vi "RunOperation.vi"(10 "Inputs":string[](array[string]), 11 "Restore in":refnum<class "Restore.lvclass">) -> (1 "Output/Failure":string, 2 "CLI Process Return Code":i32, 3 "Restore out":refnum<class "Restore.lvclass">)   [LabVIEW 2017, in "Restore.lvclass"]
uses:
  Restore.lvclass
  Restore.lvclass/Restore.ctl
  <vilib>/JKI/VIPM API/VIPM API_vipm_api.lvlib
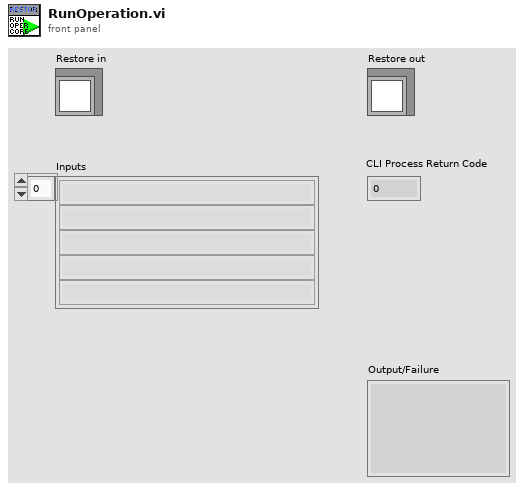
[diagram p1: front panel]
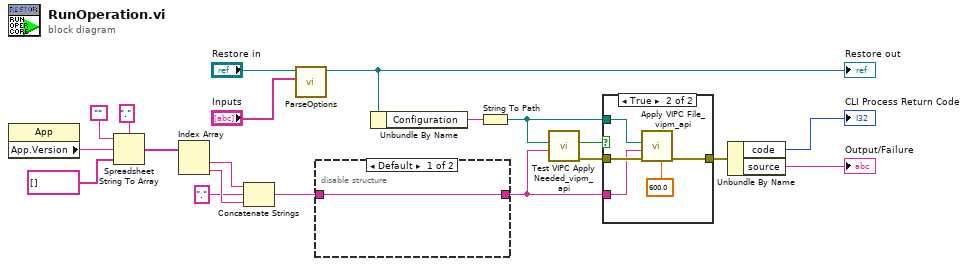
[diagram p0: block diagram]
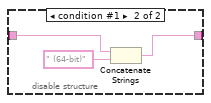
[diagram p2: hidden frame]
diagram:
  n1 = property class="App"() -> ("App.Version"=w10:string)  [unwired: 2 in, 2 out]
  n2 = Spreadsheet String To Array(delimiter (Tab)=".", format string="", spreadsheet string=w10, array type (2D Dbl)=string[] []) -> (array=w7:string[])
  n3 = Index Array(array=w7) -> (element #1=w6:string, element #2=w5:string)  [unwired: 2 in]
  n4 = Concatenate Strings(w6, "." ("string"), w5) -> (w3:string)
  n5 = call "ParseOptions.vi"("Options"="Inputs", "Restore in"="Restore in") -> ("Restore out"=w18:refnum<class "Restore.lvclass">)  [unwired: 8 in, 1 out]
  "Restore out" <- w18
  n6 = disable-structure shown="Default" {
    disable-tunnel: [w21 w23] -> w2
    disable-tunnel: w3 -> [w21 w24]
    frame condition #0 (active) {
    }
    frame condition #1 {
      n7 = Concatenate Strings(w24, " (64-bit)" ("string")) -> (w23:string)
    }
  }
  n8 = Unbundle By Name(w18) -> ("Configuration"=w17:string)
  n9 = String To Path(string=w17) -> (path=w11:path)
  n10 = call <vilib>:"Test VIPC Apply Needed_vipm_api.vi"("LabVIEW Version (use vipc version)"=w2, "VIPC File Path"=w11) -> ("error out"=w13:errorcluster, "Need to Apply?"=w12:bool)  [unwired: 7 in, 1 out]
  n11 = case shown="True" w12 {
    tunnel: [w25 w29] -> w16
    tunnel: w13 -> [w25 w28]
    tunnel: w11 -> [_ w27]
    tunnel: w2 -> [_ w26]
    frame False {
    }
    frame True {
      n12 = call <vilib>:"Apply VIPC File_vipm_api.vi"("Timeout in seconds (0: no timeout)"=600.0, "error in (no error)"=w28, "LabVIEW Version"=w26, "VIPC File"=w27) -> ("error out"=w29:errorcluster)  [unwired: 7 in]
    }
  }
  n13 = Unbundle By Name(w16) -> ("code"=→"CLI Process Return Code":i32, "source"=→"Output/Failure":string)
